vi "Actor Core.vi"(8 "error in":errorcluster, 11 "Filter Config Display in":refnum<class "Filter Config Display.lvclass">) -> (0 "error out":errorcluster, 3 "Actor out":refnum<class "Actor.lvclass">)   [LabVIEW 2017, in "Assert API Components.lvlib" / "Assert Display.lvlib" / "Filter Config Display.lvlib" / "Filter Config Display.lvclass"]
doc: "(<B>Filename</B>: Actor Framework.lvlib:Actor.lvclass:Actor Core.vi)\n\nReceives messages to the actor, reacts to them, and initiates any error handling that may shut the actor down.\n\nDescendant classes may override this VI to append parallel tasks for the actor to complete while it handles messages. Overrides use the Call Parent Method node."
uses:
  Filter Config Display.lvclass
  C:/Program Files (x86)/National Instruments/LabVIEW 2017/vi.lib/ActorFramework/Actor/Actor.lvclass
  C:/Users/ukhornp/Documents/Work/Projects/actor_assert_api/Core/Base UI Actor/Base UI Actor/Base UI Actor.lvclass
  C:/Users/ukhornp/Documents/Work/Projects/actor_assert_api/Core/Base UI Component/Base UI Component/Base UI Component.lvclass
  <vilib>/ActorFramework/Actor/Actor.lvclass
  <vilib>/ActorFramework/Actor/Actor.lvclass/Actor.ctl
  Base UI Component/Base UI Component/Base UI Component.lvclass/Base UI Component.ctl
  Base UI Actor/Base UI Actor/Base UI Actor.lvclass/Base UI Actor.ctl
  <vilib>/ActorFramework/Message Enqueuer/Message Enqueuer.lvclass/Message Enqueuer.ctl
  Filter Config Display.lvclass/Filter Config Display.ctl
  <vilib>/ActorFramework/Message Enqueuer/Init from Existing Queue.vi
  <vilib>/ActorFramework/Message Enqueuer/Enqueue.vi
  Filter Config Display Messages/Build Filter Msg/Build Filter Msg.lvclass
  C:/Program Files (x86)/National Instruments/LabVIEW 2017/vi.lib/ActorFramework/Message/Message.lvclass
  Assert Display/Assert Display Messages/Launch Dynamic Filter Window PT Msg/Launch Dynamic Filter Window PT Msg.lvclass
  <vilib>/Utility/LVClass/Get LV Class Name.vi
  <resource>/AFDebug/Generate Trace for Message.vi
  <vilib>/ActorFramework/Message Priority Queue/Priority Enqueue.vi
  Base UI Component/Base UI Component/Base UI Component.lvclass
  <vilib>/ActorFramework/Message Enqueuer/Message Enqueuer.lvclass
  Base UI Actor/Base UI Actor/Base UI Actor.lvclass
panel:
  in  "Dynamic Filter Window":bool
  in  "Filters":i32(listbox)
  in  "New Filter":bool
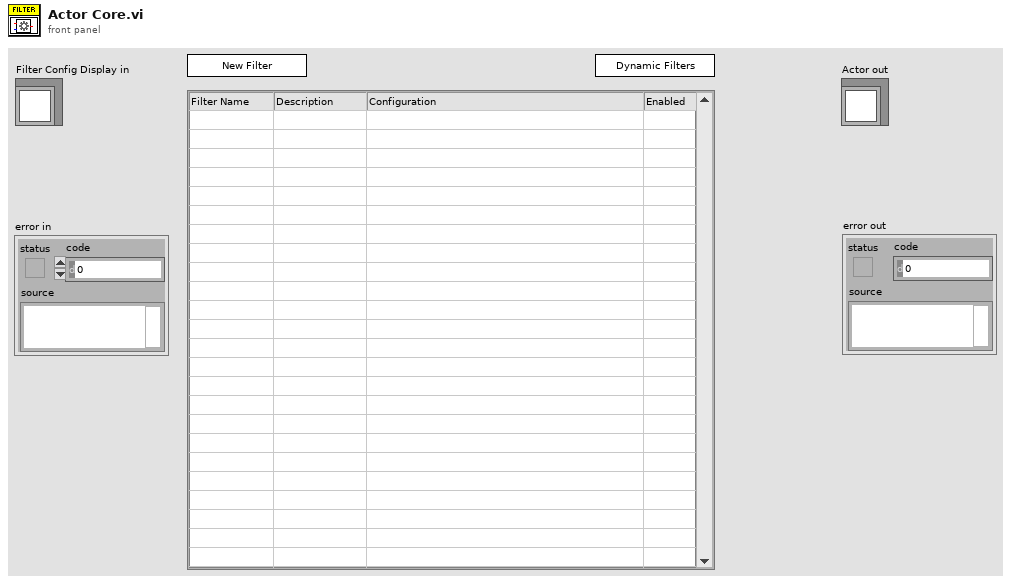
[diagram p1: front panel]
types:
  T1 = typedef "LVPoint32TypeDef.ctl" = cluster{"Horizontal":i32, "Vertical":i32}
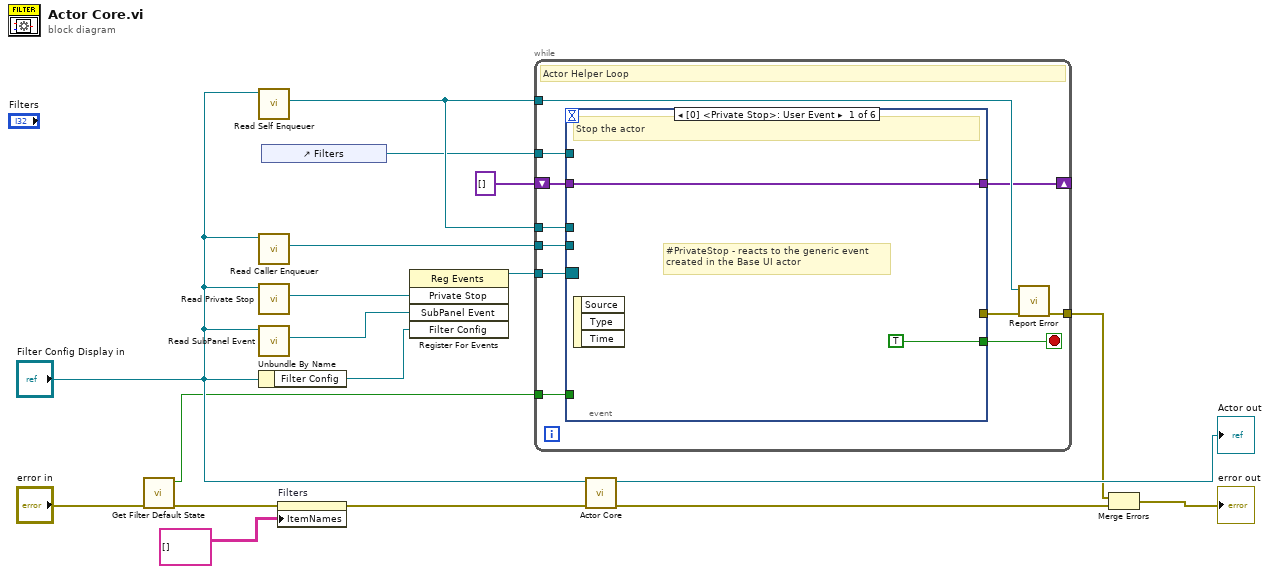
[diagram p0: block diagram]
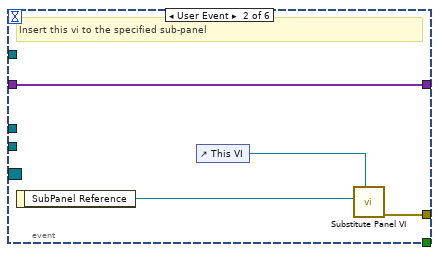
[diagram p2: hidden frame]
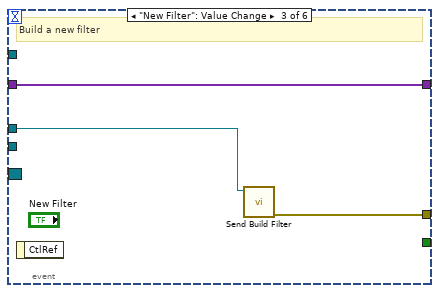
[diagram p3: hidden frame]
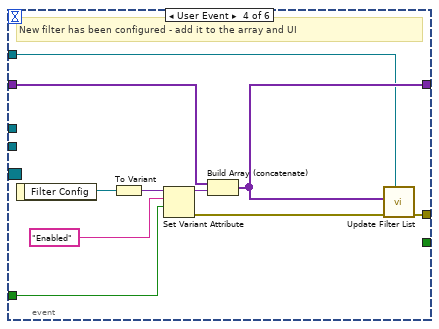
[diagram p4: hidden frame]
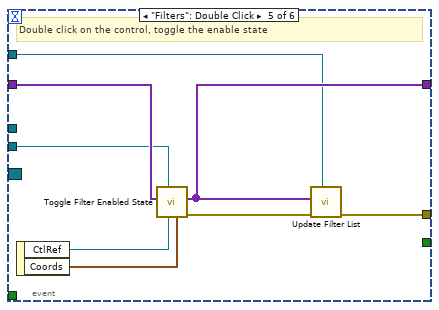
[diagram p5: hidden frame]
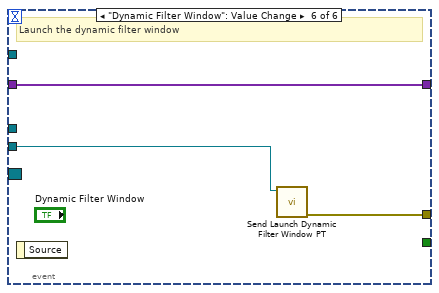
[diagram p6: hidden frame]
diagram:
  n1 = call "Get Filter Default State.vi"("error in (no error)"="error in") -> ("error out"=w3:errorcluster, "Filters Enabled By Default?"=w2:bool)  [unwired: 9 in]
  n2 = call <vilib>:"Read Self Enqueuer.vi"("Actor"="Filter Config Display in") -> ("Self Enqueuer"=w10:refnum<class "Message Enqueuer.lvclass">)  [unwired: 10 in]
  n3 = call <vilib>:"Read Caller Enqueuer.vi"("Actor"="Filter Config Display in") -> ("Caller Enqueuer"=w9:refnum<class "Message Enqueuer.lvclass">)  [unwired: 10 in]
  n4 = call "Read Private Stop.vi"("Base UI Actor in"="Filter Config Display in") -> ("Private Stop"=w15:refnum<user-event>)  [unwired: 10 in]
  n5 = call "Read SubPanel Event.vi"("Base UI Component in"="Filter Config Display in") -> ("SubPanel Event"=w14:refnum<user-event>)  [unwired: 10 in]
  n6 = Unbundle By Name("Filter Config Display in") -> ("Filter Config"=w7:refnum<user-event>)
  n7 = control-ref of="Filters"() -> (w1:refnum<vi>)
  n8 = property on="Filters" class="MCListbox (strict)"(error in=w3, "ItemNames"=string[][] [] ("Item Names")) -> (error out=w5:errorcluster)  [unwired: 1 in, 1 out]
  n9 = register-events(w15, w14, w7) -> (reference out=w13:refnum<event-registration>)  [unwired: 2 in, 1 out]
  n10 = while {
    tunnel: w13 -> [w29]
    tunnel: [w26] -> w11
    tunnel: w10 -> [w25]
    tunnel: w10 -> [w24]
    tunnel: w9 -> [w23]
    shift-right: [w21] -> _
    shift-left: variant[] [] ("Array") -> [w22]
    tunnel: w2 -> [w20]
    tunnel: w1 -> [w19]
    stop <- w27 stop-if-true
    # "Actor Helper Loop"
    n11 = event shown="[0] <Private Stop>: User Event" {
      selector: w29 -> [_ _ _ _ _ _]
      dyn-events: _ -> [_ _ _ _ _ _]
      timeout: _ -> [_ _ _ _ _ _]
      tunnel: [_ w35 w37 w48 w55 w59] -> w28
      tunnel: [TRUE _ _ _ _ _] -> w27
      tunnel: w24 -> [_ _ w38 _ _ _]
      tunnel: w23 -> [_ _ _ _ w51 w58]
      tunnel: w22 -> [w30 w32 w36 w47 w54 w57]
      tunnel: [w30 w32 w36 w46 w50 w57] -> w21
      tunnel: w20 -> [_ _ _ w41 _ _]
      tunnel: w19 -> [_ _ _ w39 w49 _]
      event User Event {
        # "#PrivateStop - reacts to the generic event created in the Base UI actor"
        # "Stop the actor"
        n12 = event-data() -> ()  [unwired: 1 in, 3 out]
      }
      event User Event {
        # "Insert this vi to the specified sub-panel"
        n13 = event-data() -> ("SubPanel Reference"=w34:refnum<vi>)  [unwired: 1 in]
        n14 = control-ref of="This VI"() -> (w33:refnum<vi>)
        n15 = call "Substitute Panel VI.vi"("VI Reference"=w33, "SubPanel Reference"=w34) -> ("error out"=w35:errorcluster)  [unwired: 9 in]
      }
      event "New Filter": Value Change {
        # "Build a new filter"
        n16 = event-data() -> ()  [unwired: 1 in, 1 out]
        n17 = call "Send Build Filter.vi"("Message Enqueuer"=w38) -> ("error out"=w37:errorcluster)  [unwired: 9 in, 1 out]
      }
      event User Event {
        # "New filter has been configured - add it to the array and UI"
        n18 = event-data() -> ("Filter Config"=w45:refnum<class "Base Filter.lvclass">)  [unwired: 1 in]
        n19 = To Variant(anything=w45) -> (Variant=w44:variant)
        n20 = Set Variant Attribute(Variant=w44, name="Enabled", value=w41) -> (Variant out=w43:variant, error out=w40:errorcluster)  [unwired: 1 in, 1 out]
        n21 = Build Array (concatenate)(w47, w43) -> (w46:variant[])
        n22 = call "Update Filter List.vi"("MCListbox Refnum"=w39, "error in (no error)"=w40, "Filter Array"=w46) -> ("error out"=w48:errorcluster)  [unwired: 8 in]
      }
      event "Filters": Double Click {
        # "Double click on the control, toggle the enable state"
        n23 = event-data() -> ("CtlRef"=w53:refnum<vi>, "Coords"=w52:T1)  [unwired: 1 in]
        n24 = call "Toggle Filter Enabled State.vi"("Click Coordinates"=w52, "MulticolumnListbox in"=w53, "Caller Enqueuer"=w51, "Filter Array in"=w54) -> ("error out"=w56:errorcluster, "Filter Array out"=w50:variant[])  [unwired: 6 in]
        n25 = call "Update Filter List.vi"("MCListbox Refnum"=w49, "error in (no error)"=w56, "Filter Array"=w50) -> ("error out"=w55:errorcluster)  [unwired: 8 in]
      }
      event "Dynamic Filter Window": Value Change {
        # "Launch the dynamic filter window"
        n26 = event-data() -> ()  [unwired: 1 in, 1 out]
        n27 = call "Send Launch Dynamic Filter Window PT.vi"("Message Enqueuer"=w58) -> ("error out"=w59:errorcluster)  [unwired: 9 in, 1 out]
      }
    }
    n28 = call "Report Error.vi"("error in (no error)"=w28, "Self Enqueuer"=w25) -> ("error out"=w26:errorcluster)  [unwired: 9 in]
  }
  n29 = call-parent "Actor Core.vi"("error in"=w5, "Actor in"="Filter Config Display in") -> ("error out"=w18:errorcluster, "Actor out"=→"Actor out":refnum<class "Actor.lvclass">)  [unwired: 8 in]
  n30 = Merge Errors(w11, w18) -> (→"error out":errorcluster)
